vi "CheckOldFileName.vi"(10 "Filename":string, 11 "Folder":path) -> (3 "path":path)   [LabVIEW 2024]
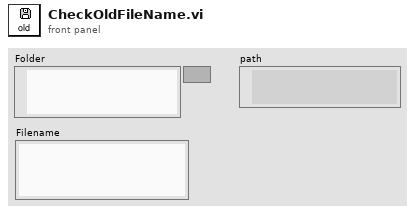
[diagram p1: front panel]
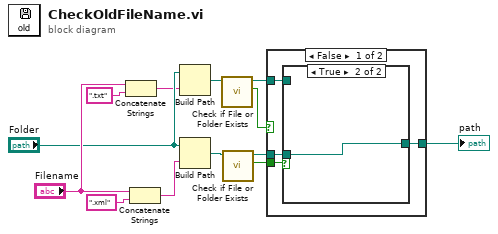
[diagram p0: block diagram]
diagram:
  n1 = Concatenate Strings("Filename", ".txt" ("name or relative path")) -> (w7:string)
  n2 = Concatenate Strings("Filename", ".xml" ("name or relative path")) -> (w12:string)
  n3 = Build Path(base path="Folder", name or relative path=w7) -> (appended path=w9:path)
  n4 = Build Path(base path="Folder", name or relative path=w12) -> (appended path=w6:path)
  n5 = call <vilib>:"Check if File or Folder Exists.vi"("path"=w9) -> ("file or folder exists?"=w5:bool, "dup path"=w3:path)  [unwired: 8 in, 1 out]
  n6 = call <vilib>:"Check if File or Folder Exists.vi"("path"=w6) -> ("file or folder exists?"=w2:bool, "dup path"=w1:path)  [unwired: 8 in, 1 out]
  n7 = case shown="False" w5 {
    tunnel: [w16 w20] -> w4
    tunnel: w3 -> [w14 w20]
    tunnel: w2 -> [w17 _]
    tunnel: w1 -> [w15 _]
    frame False {
      n8 = case shown="True" w17 {
        tunnel: [w18 w19] -> w16
        tunnel: w15 -> [_ w19]
        tunnel: w14 -> [w18 _]
        frame False {
        }
        frame True {
        }
      }
    }
    frame True {
    }
  }
  "path" <- w4
